vi "Rh_to_Absolute_Humidity.vi"(1 "Temperature (F)":dbl, 2 "Relative Humidity":dbl) -> (0 "Absolute Humidity":dbl)   [LabVIEW 2020]
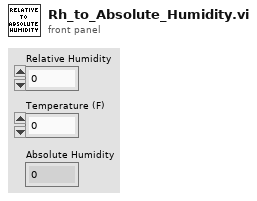
[diagram p1: front panel]
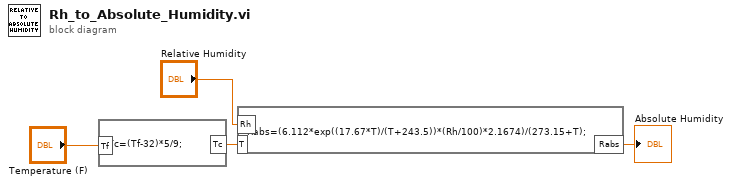
[diagram p0: block diagram]
diagram:
  n1 = formula code="Tc=(Tf-32)*5/9;"("Tf"="Temperature (F)") -> ("Tc"=w2:dbl)
  n2 = formula code="Rabs=(6.112*exp((17.67*T)/(T+243.5))*(Rh/100)*2.1674)/(273.15+T);"("Rh"="Relative Humidity", "T"=w2) -> ("Rabs"=→"Absolute Humidity":dbl)
